vi "Initialize.vi"(8 "error in (no error)":errorcluster, 9 "Reset (True)":bool, 10 "ID Query (True)":bool=TRUE, 11 "VISA resource name":refnum<visa-resource-name>="COM37") -> (0 "error out":errorcluster, 3 "VISA resource name out":refnum<visa-resource-name>="COM37")   [LabVIEW 2014, in "YbTempCtrl.lvlib"]
doc: "Establishes communication with the instrument and optionally performs an instrument identification query and/or an instrument reset. It also places the instrument in a default state needed for other instrument driver operations. Therefore, call this VI before calling other instrument driver VIs for this instrument. Generally, you need to call the <b>Initialize</b> VI only once at the beginning of an application."
uses:
  YbTempCtrl.lvlib
panel:
  in  "Expected version":string="v4.3"
  out "ID Response":string="v4.2\r\n"
  # "(c) 2015 NPL.  ALL RIGHTS RESERVED."
  # "EDIT: Change control description to remove example text for buses not supported."
  # "EDIT: Serial settings must match those on the physical instrument.  Review user's manual to determine the correct Flow Control protocol for the instrument.  \"None\" is the least robust option for this setting, and could lead to unreliable data transmission."
  # "EDIT: If your instrument does not support ID query or Reset, remove the ID Query or Reset control from the front panel and delete the case structure with the ID Query or Reset code from the block diagram."
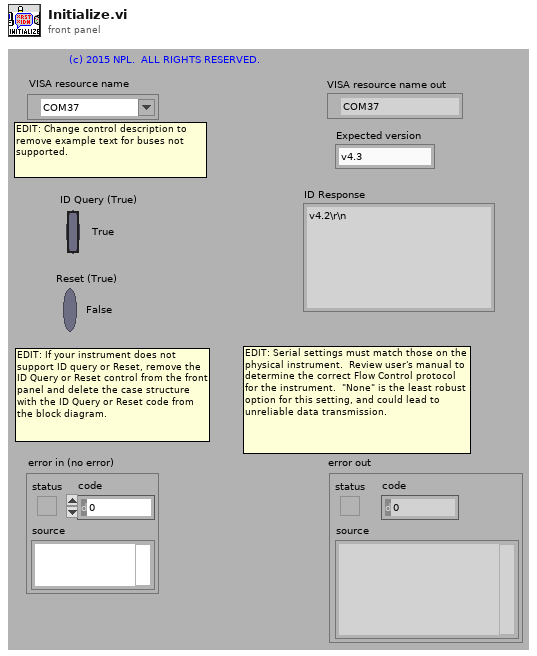
[diagram p1: front panel]
types:
  T1 = cluster{"Baud Rate":u32, "Parity":u16, "Data Bits":u16, "Stop Bits":u16, "Flow Control":u16}
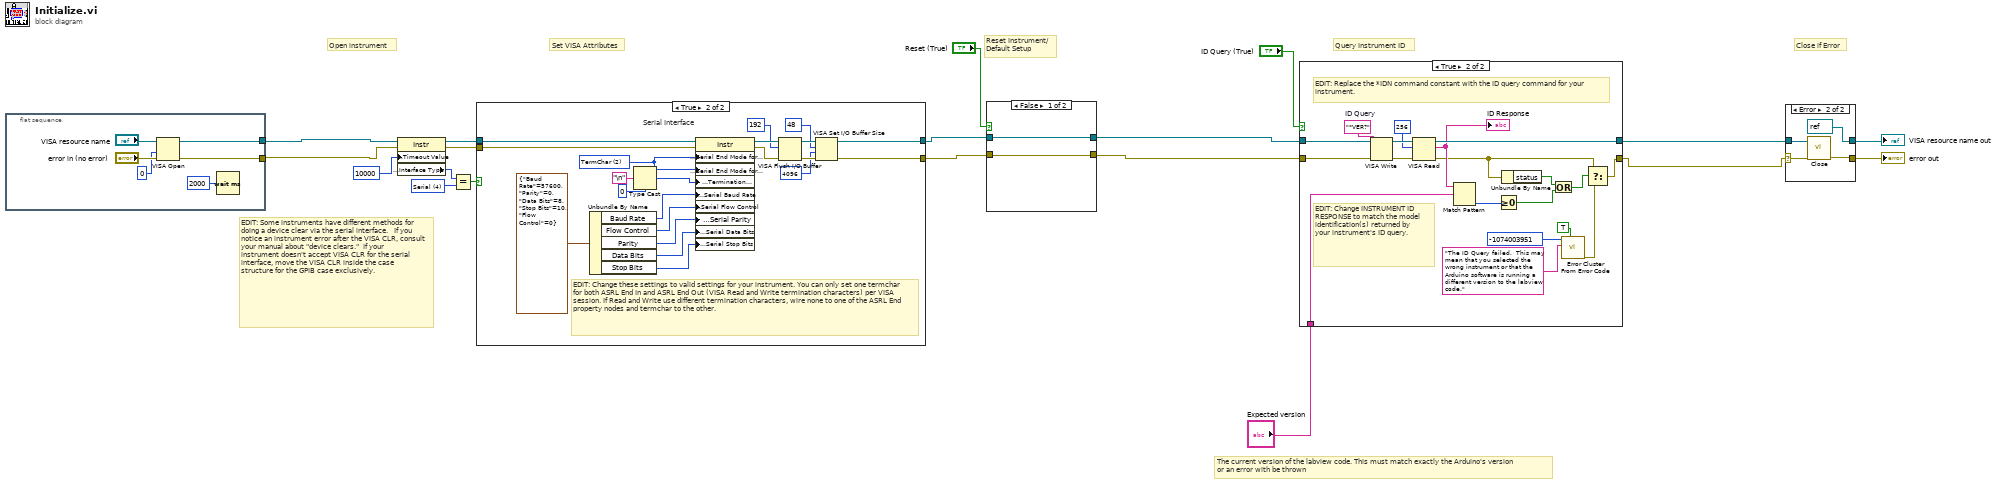
[diagram p0: block diagram]
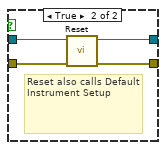
[diagram p3: hidden frame]
diagram:
  w13 = u16 4 items=["GPIB"=1, "VXI"=2, "GPIB-VXI"=3, "Serial"=4, "PXI"=5, "TCPIP"=6, "USB"=7] ("Interface Information:Interface Type")
  # "The current version of the labview code. This must match exactly the Arduino's version\nor an error with be thrown"
  # "Close if Error"
  # "Reset Instrument/\nDefault Setup"
  # "EDIT: Some instruments have different methods for doing a device clear via the serial interface.   If you notice an instrument error after the VISA CLR, consult your manual about \"device clears.\"  If your instrument doesn't accept VISA CLR for the serial interface, move the VISA CLR inside the case  structure for the GPIB case exclusively."
  # "Set VISA Attributes"
  # "Query Instrument ID"
  # "Open instrument"
  n1 = flat-sequence {
    tunnel: [w22] -> w6
    tunnel: [w21] -> w7
    frame #0 {
      n2 = VISA Open(access mode=u32 0, error in (no error)="error in (no error)", VISA resource name="VISA resource name") -> (VISA resource name=w22:refnum<visa-resource-name>, error out=w21:errorcluster)  [unwired: 2 in]
      n3 = Wait (ms)(milliseconds to wait=u32 2000) -> ()  [unwired: 1 out]
    }
  }
  n4 = property class="Instr"(reference=w6, error in=w7, "General Settings:Timeout Value"=u32 10000) -> (reference out=w16:refnum<visa-resource-name>, error out=w15:errorcluster, "Interface Information:Interface Type"=w18:u16)
  n5 = Equal?(x=w18, y=w13) -> (x = y?=w14:bool)
  n6 = case shown="True" w14 {
    tunnel: [w26 w29] -> w8
    tunnel: [w27 w28] -> w9
    tunnel: w16 -> [w26 w47]
    tunnel: w15 -> [w27 w48]
    frame False {
      # "EDIT: Remove interfaces not supported by your instrument."
      # "GPIB, TCP/IP, and USB Interface"
    }
    frame True {
      w37 = u16 2 items=["None", "LastBit", "TermChar"] ("Serial Settings:Serial End Mode for Reads")
      # "EDIT: Change these settings to valid settings for your instrument. You can only set one termchar for both ASRL End In and ASRL End Out (VISA Read and Write termination characters) per VISA session. If Read and Write use different termination characters, wire none to one of the ASRL End property nodes and termchar to the other."
      # "Serial Interface"
      n7 = Unbundle By Name(T1 {"Baud Rate"=57600, "Parity"=0, "Data Bits"=8, "Stop Bits"=10, "Flow Control"=0} ("Serial Configuration")) -> ("Baud Rate"=w35:u32, "Flow Control"=w31:u16, "Parity"=w33:u16, "Data Bits"=w34:u16, "Stop Bits"=w30:u16)
      n8 = Type Cast(type=u8 0, x="\n" ("Line Feed Constant")) -> (*(type *) &x=w36:u8)
      n9 = property class="Instr"(reference=w47, error in=w48, "Serial Settings:Serial End Mode for Reads"=w37, "Serial Settings:Serial End Mode for Writes"=w37, "Message Based Settings:Termination Character"=w36, "Serial Settings:Serial Baud Rate"=w35, "Serial Settings:Serial Flow Control"=w31, "Serial Settings:Serial Parity"=w33, "Serial Settings:Serial Data Bits"=w34, "Serial Settings:Serial Stop Bits"=w30) -> (reference out=w43:refnum<visa-resource-name>, error out=w45:errorcluster)
      n10 = VISA Flush I/O Buffer(VISA resource name=w43, mask (16)=u16 192, error in (no error)=w45) -> (VISA resource name out=w46:refnum<visa-resource-name>, error out=w44:errorcluster)
      n11 = VISA Set I/O Buffer Size(VISA resource name=w46, mask (16)=u16 48, size (4096)=u32 4096 ("size (0)"), error in (no error)=w44) -> (VISA resource name out=w29:refnum<visa-resource-name>, error out=w28:errorcluster)
    }
  }
  n12 = case shown="False" "Reset (True)" {
    tunnel: w9 -> [w49 w51]
    tunnel: [w49 w54] -> w4
    tunnel: w8 -> [w50 w52]
    tunnel: [w50 w53] -> w5
    frame False {
    }
    frame True {
      # "Reset also calls Default Instrument Setup"
      n13 = call "Reset.vi"("error in (no error)"=w51, "VISA resource name"=w52) -> ("error out"=w54:errorcluster, "VISA resource name out"=w53:refnum<visa-resource-name>)  [unwired: 8 in]
    }
  }
  n14 = case shown="True" "ID Query (True)" {
    tunnel: [w55 w75] -> w3
    tunnel: [w56 w72] -> w2
    tunnel: w5 -> [w56 w73]
    tunnel: w4 -> [w55 w74]
    tunnel: "Expected version" -> [_ w57]
    frame False {
    }
    frame True {
      w67 = "*VER?"  # ID Query
      # "EDIT: Replace the *IDN command constant with the ID query command for your instrument."
      # "EDIT: Change INSTRUMENT ID RESPONSE to match the model identification(s) returned by your instrument's ID query."
      n15 = VISA Write(VISA resource name=w73, write buffer=w67, error in (no error)=w74) -> (VISA resource name out=w70:refnum<visa-resource-name>, error out=w69:errorcluster)  [unwired: 1 out]
      n16 = VISA Read(VISA resource name=w70, byte count=u32 256, error in (no error)=w69) -> (VISA resource name out=w72:refnum<visa-resource-name>, read buffer=w71:string, error out=w61:errorcluster)  [unwired: 1 out]
      "ID Response" <- w71
      n17 = Match Pattern(string=w71, regular expression=w57) -> (offset past match=w62:i32)  [unwired: 1 in, 3 out]
      n18 = Greater Or Equal To 0?(x=w62) -> (x >= 0?=w59:bool)
      n19 = Unbundle By Name(w61) -> ("status"=w60:bool)
      n20 = Or(x=w60, y=w59) -> (x .or. y?=w58:bool)
      n21 = call <vilib>:"Error Cluster From Error Code.vi"("show call chain? (False)"=TRUE, "error message (\"\")"="The ID Query failed.  This may mean that you selected the wrong instrument or that the Arduino software is running a different version to the labview code." ("Source (VI Name)"), "error code (0)"=-1074003951 ("Code")) -> ("error out"=w66:errorcluster)  [unwired: 6 in]
      n22 = Select(t=w61, s=w58, f=w66) -> (s? t:f=w75:errorcluster)
    }
  }
  n23 = case shown="Error" w3 {
    selector: w3 -> [w76 w79]
    tunnel: w2 -> [w77 w80]
    tunnel: [w77 refnum<visa-resource-name> refnum ("VISA resource name out")] -> w12
    tunnel: [w76 w78] -> w11
    frame No Error {
    }
    frame Error {
      n24 = call "Close.vi"("error in (no error)"=w79, "VISA resource name"=w80) -> ("error out"=w78:errorcluster)  [unwired: 9 in]
    }
  }
  "VISA resource name out" <- w12
  "error out" <- w11
